vi "Action Point_Close.vi"(8 "error in":errorcluster, 11 "Action Point in":refnum<class "Action Point.lvclass">) -> (0 "error out":errorcluster, 3 "Action Point out":refnum<class "Action Point.lvclass">)   [LabVIEW 2025, in "Action Point.lvclass"]
uses:
  Action Point.lvclass
  Interfaces/IUnmanaged/IUnmanaged.lvclass
  Action Point.lvclass/Action Point.ctl
  Interfaces/ILog Data/ILog Data.lvclass
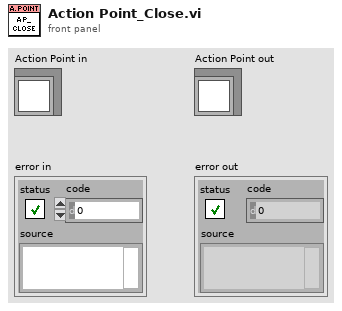
[diagram p1: front panel]
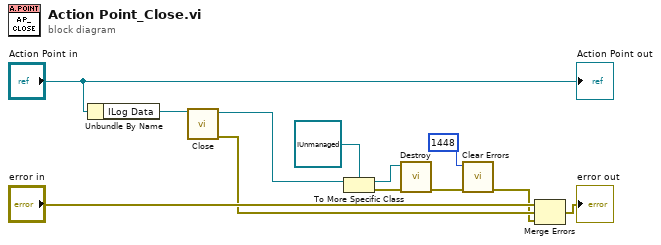
[diagram p0: block diagram]
diagram:
  n1 = Unbundle By Name("Action Point in") -> ("ILog Data"=w11:refnum<class "ILog Data.lvclass">)
  n2 = call-dynamic "Close.vi"("IClose in"=w11) -> ("error out"=w6:errorcluster, "IClose out"=w9:refnum<class "ILog Data.lvclass">)  [unwired: 9 in]
  n3 = To More Specific Class(target class=refnum<class "IUnmanaged.lvclass"> refnum ("IUnmanaged.lvclass"), reference=w9) -> (specific class reference=w3:refnum<class "IUnmanaged.lvclass">, error out=w8:errorcluster)  [unwired: 1 in]
  n4 = call-dynamic "Destroy.vi"("error in"=w8, "IUnmanaged in"=w3) -> ("error out"=w5:errorcluster)  [unwired: 8 in, 1 out]
  n5 = call <vilib>:"Clear Errors.vi"("error in (no error)"=w5, "specific error code to clear (0: all)"=1448) -> ("error out"=w2:errorcluster)  [unwired: 4 in, 1 out]
  n6 = Merge Errors("error in", w6, w2) -> (→"error out":errorcluster)
  "Action Point out" <- "Action Point in"
